vi "PH_GetBBInformation.PC Get Info.vi"(2 "MCL Listbox GUI Ref":refnum<vi>, 5 "error in":errorcluster) -> (19 "error out":errorcluster)   [LabVIEW 2014, in "PH_GetBBInformation.lvlib"]
doc: "This is the proc case \"get information\"."
uses:
  PH_GetBBInformation.lvlib
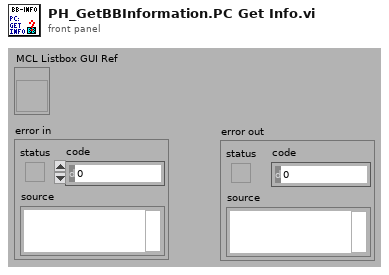
[diagram p1: front panel]
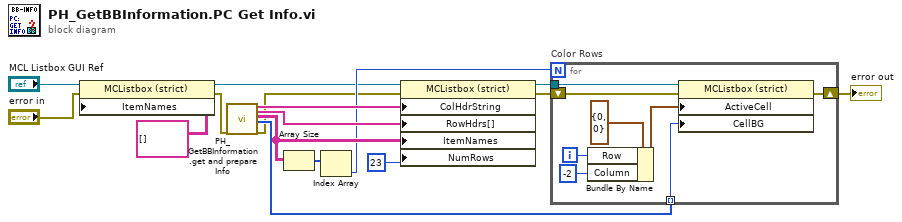
[diagram p0: block diagram]
diagram:
  n1 = property class="MCListbox (strict)"(reference="MCL Listbox GUI Ref", error in="error in", "ItemNames"=string[][] [] ("Value")) -> (reference out=w6:refnum<vi>, error out=w4:errorcluster)
  n2 = call "PH_GetBBInformation.get and prepare Info.vi"("error in"=w4) -> ("ColHdrs[]"=w13:string[], "RowHdrs[]"=w15:string[], "ItemNames"=w16:string[][], "Row Cell BG"=w14:u32[], "error out"=w2:errorcluster)  [unwired: 14 in]
  n3 = Array Size(array=w16) -> (size(s)=w12:i32[])
  n4 = Index Array(array=w12) -> (element=w8:i32)  [unwired: 1 in]
  n5 = property class="MCListbox (strict)"(reference=w6, error in=w2, "ColHdrString"=w13, "RowHdrs[]"=w15, "ItemNames"=w16, "NumRows"=u32 23 ("Number of Rows")) -> (reference out=w9:refnum<vi>, error out=w10:errorcluster)
  n6 = for "Color Rows" {
    N: w8 -> [_]
    tunnel: w9 -> [w22]
    shift-right: [w23] -> w1
    shift-left: w10 -> [w24]
    tunnel: w14 -> [w19] mode=indexing
    i -> [w18]
    n7 = Bundle By Name(cluster=cluster{"Row":i32, "Column":i32} {"Row"=0, "Column"=0} ("Active Cell:Active Cell"), "Row"=w18, "Column"=-2 ("Row")) -> (w21:cluster{"Row":i32, "Column":i32})
    n8 = property class="MCListbox (strict)"(reference=w22, error in=w24, "ActiveCell"=w21, "CellBG"=w19) -> (error out=w23:errorcluster)  [unwired: 1 out]
  }
  "error out" <- w1
